vi "Impedance tube v1.0.0.vi"() -> ()   [LabVIEW 2021]
uses:
  <vilib>/Analysis/1siggen.llb/Ramp Pattern by Samples.vi
  <vilib>/express/express analysis/Spectral/Block/exnSpectralBlock spectral measurements RMS poly.vi
  <vilib>/express/express analysis/Spectral/Block/exnSpectralBlock spectral measurements RMS DDT.vi
  <vilib>/express/express arith-compare/Formula/XNode/ExpressFormulaBlockNode.xnode
  <vilib>/express/express analysis/Spectral/XNode/ExpressSpectralMeasurementsBlockNode.xnode
  <vilib>/Analysis/NI_AALPro.lvlib
  <vilib>/Analysis/NI_AALBase.lvlib
panel:
  out "Probe":dbl[](graph)
  out "Rr":dbl[](graph)
  out "Absorption coeff":dbl[](graph)
  in  "number of samples":i32=2048
  out "MIC 2":dynamicdata(graph)
  out "MIC 2":dbl
  out "FFT1":dynamicdata(graph)
  out "MIC 1":dynamicdata(graph)
  out "MIC 1":dbl
  in  "stop (F)":bool
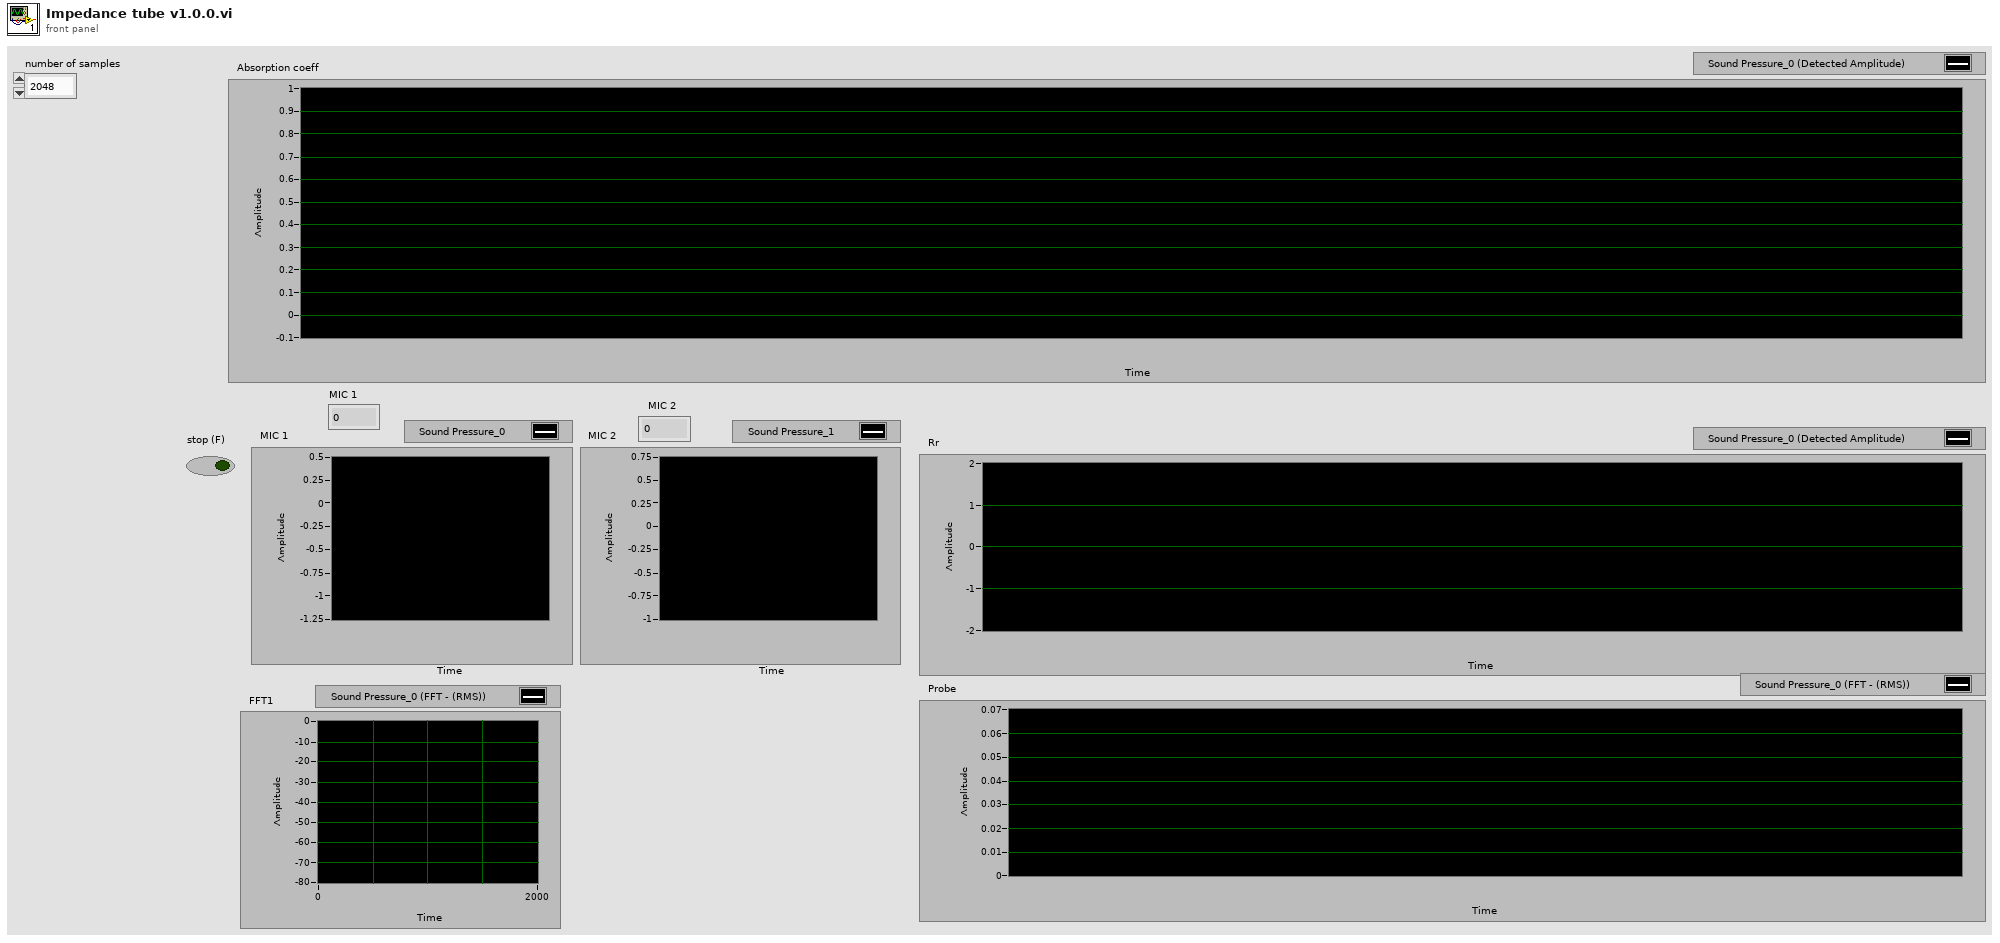
[diagram p1: front panel]
types:
  T1 = cluster{"averaging mode":u16, "weighting mode":u16, "number of averages":u32}
  T2 = cluster{"dB On (F)":bool, "unwrap phase (F)":bool, "convert to degree (F)":bool}
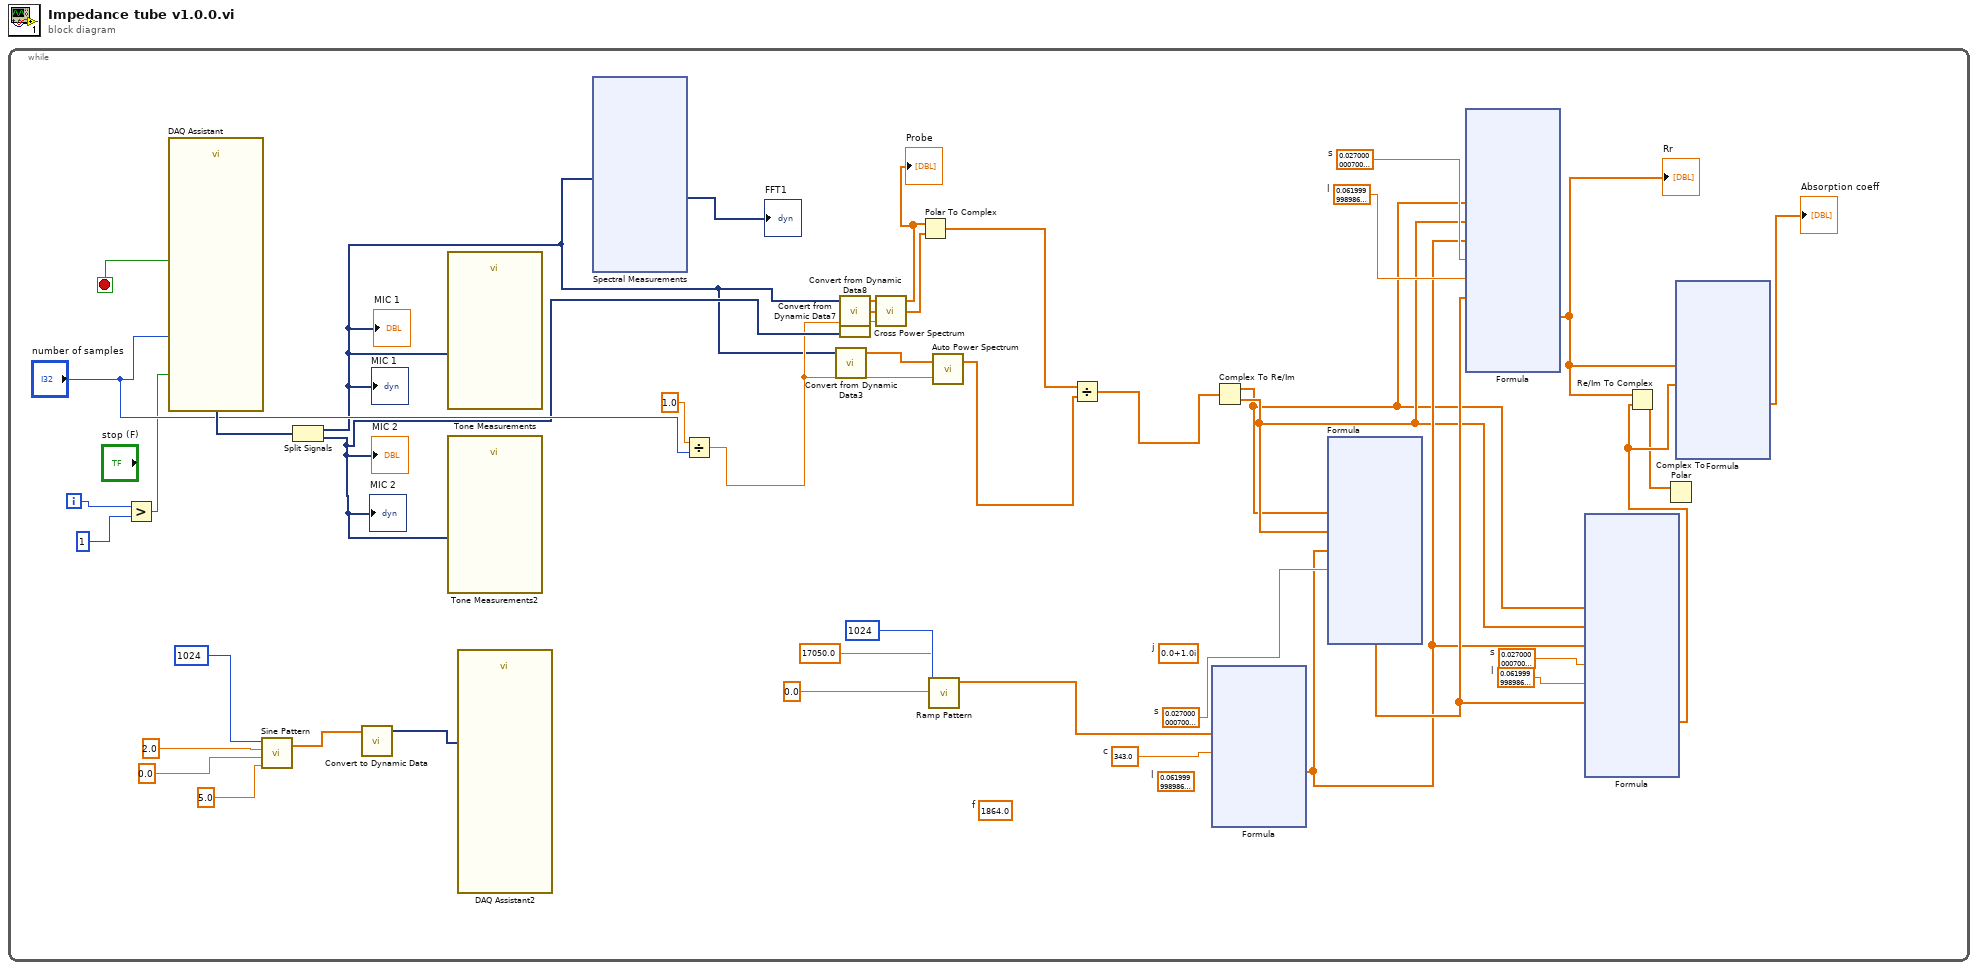
[diagram p0: block diagram]
diagram:
  n1 = while {
    i -> [w31]
    stop <- w43 stop-if-true
    w36 = sgl 0.062  # l
    w37 = sgl 0.027  # s
    w38 = sgl 0.062  # l
    w39 = sgl 0.027  # s
    (unwired) sgl 0.062  # l
    (unwired) sgl 1864.0  # f
    w40 = sgl 0.027  # s
    w41 = sgl 343.0  # c
    (unwired) csg 0.0+1.0i  # j
    n2 = Greater?(x=w31, y=1) -> (0:w24:bool)
    n3 = call "DAQ Assistant"("number of samples"="number of samples", "stop (F)"=w24) -> ("data"=w42:dynamicdata, "stopped"=w43:bool)  [unwired: 14 in, 2 out]
    n4 = call <vilib>:"Sine Pattern.vi"("cycles"=5.0, "phase(degrees)"=0.0, "amplitude"=2.0, "samples"=1024) -> ("Sinusoidal Pattern"=w6:dbl[])  [unwired: 1 out]
    n5 = Split Signals(w42) -> (w16:dynamicdata, w21:dynamicdata)  [unwired: 2 in]
    "MIC 1" <- w16
    "MIC 1" <- w16
    "MIC 2" <- w21
    "MIC 2" <- w21
    n6 = call "Convert to Dynamic Data"("Array"=w6) -> ("Dynamic Data Type"=w5:dynamicdata)  [unwired: 3 in]
    n7 = call "Tone Measurements"("Signals"=w16) -> ()  [unwired: 8 in, 3 out]
    n8 = call "Tone Measurements2"("Signals"=w21) -> ()  [unwired: 8 in, 3 out]
    n9 = call "DAQ Assistant2"("data"=w5) -> ()  [unwired: 16 in, 3 out]
    n10 = xnode "Spectral Measurements"("Signals"=w16) -> ("FFT - (RMS)"=→"FFT1":dynamicdata)  [unwired: 1 in, 2 out]
    n11 = Divide(x=1.0, y="number of samples") -> (x/y=w18:dbl)
    n12 = call "Convert from Dynamic Data3"("Dynamic Data Type"=w16) -> ("Array"=w15:dbl[])  [unwired: 3 in]
    n13 = call "Convert from Dynamic Data7"("Dynamic Data Type"=w16) -> ("Array"=w22:dbl[])  [unwired: 3 in]
    n14 = call "Convert from Dynamic Data8"("Dynamic Data Type"=w21) -> ("Array"=w20:dbl[])  [unwired: 3 in]
    n15 = call <vilib>:"Cross Power Spectrum.vi"("dt"=w18, "Signal Y (V)"=w20, "Signal X (V)"=w22) -> ("Cross Power XY Spectrum Phase (radians)"=w19:dbl[], "Cross Power XY Spectrum Mag (V^2rms)"=w17:dbl[])  [unwired: 1 out]
    "Probe" <- w17
    n16 = Polar To Complex(1:w19, 2:w17) -> (0:w14:cdb[])
    n17 = call-poly <vilib>:"Ramp Pattern.vi"("start"=0.0, "end"=17050.0, "samples"=1024) -> ("Ramp Pattern"=w7:dbl[])  [unwired: 7 in, 1 out]
    n18 = call <vilib>:"Auto Power Spectrum.vi"("dt"=w18, "Signal (V)"=w15) -> ("Power Spectrum (V^2 rms)"=w13:dbl[])  [unwired: 1 out]
    n19 = Divide(x=w14, y=w13) -> (x/y=w12:cdb[])
    n20 = xnode "Formula"("f"=w7, "c"=w41) -> ("Result"=w34:dbl[])  [unwired: 1 in, 1 out]
    n21 = Complex To Re/Im(x + iy=w12) -> (x=w28:dbl[], y=w33:dbl[])
    n22 = xnode "Formula"("Hr"=w28, "Hi"=w33, "k"=w34, "s"=w40) -> ("Result"=w35:dbl[])  [unwired: 1 in, 1 out]
    n23 = xnode "Formula"("Hr"=w28, "Hi"=w33, "k"=w34, "s"=w39, "l"=w38, "D"=w35) -> ("Result"=w25:dbl[])  [unwired: 1 in, 1 out]
    "Rr" <- w25
    n24 = xnode "Formula"("Hr"=w28, "Hi"=w33, "k"=w34, "s"=w37, "l"=w36, "D"=w35) -> ("Result"=w32:dbl[])  [unwired: 1 in, 1 out]
    n25 = Re/Im To Complex(1:w32, 2:w25) -> (0:w29:cdb[])
    n26 = Complex To Polar(r * e^(i*theta)=w29) -> ()  [unwired: 2 out]
    n27 = xnode "Formula"("Rr"=w25, "Ri"=w32) -> ("Result"=→"Absorption coeff":dbl[])  [unwired: 1 in, 1 out]
  }
